vi "Get_FIFO.vi"(8 "error in (no error)":errorcluster) -> (0 "error out":errorcluster, 2 "TrajectoryFIFO":T1)   [LabVIEW 2019, in "Kinova MICO² USB.lvlib"]
uses:
  <vilib>/Utility/error.llb/Error Cluster From Error Code.vi
  <vilib>/ErrorRing/Error Ring.xnode
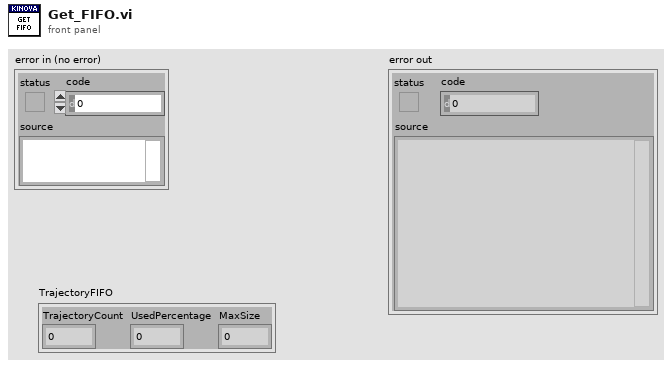
[diagram p1: front panel]
types:
  T1 = cluster{"TrajectoryCount":u32, "UsedPercentage":sgl, "MaxSize":u32}
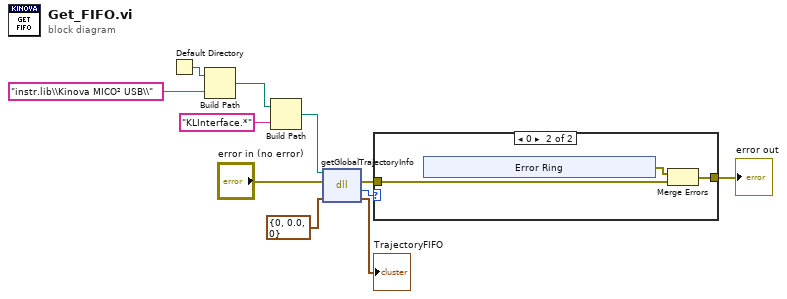
[diagram p0: block diagram]
diagram:
  n1 = Default Directory() -> (w3:path)
  n2 = Build Path(base path=w3, name or relative path="instr.lib\\Kinova MICO² USB\\") -> (appended path=w1:path)
  n3 = Build Path(base path=w1, name or relative path="KLInterface.*") -> (appended path=w5:path)
  n4 = dll-call lib="C:/Users/mcjssdcc/Documents/Kinova-Labview-Interface/KLInterface.dll" fn="getGlobalTrajectoryInfo"(path in=w5, error in="error in (no error)", "point"=T1 {"TrajectoryCount"=0, "UsedPercentage"=0.0, "MaxSize"=0} ("TrajectoryFIFO")) -> (error out=w10:errorcluster, "return type"=w9:i32, "point"=→"TrajectoryFIFO":T1)  [unwired: 1 in, 1 out]
  n5 = case shown="0" w9 {
    tunnel: [w12 w14] -> w8
    tunnel: w10 -> [w12 w13]
    frame 1, Default {
    }
    frame 0 {
      n6 = xnode "Error Ring"() -> ("error out"=w15:errorcluster)
      n7 = Merge Errors(w15, w13) -> (w14:errorcluster)
    }
  }
  "error out" <- w8
